vi "Open.vi"   [LabVIEW 2011, in "LMH-Xbox-One-Controller.lvlib"]
uses:
  LMH-Xbox-One-Controller.lvlib
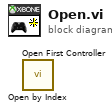
[diagram p0: block diagram]
diagram:
  n1 = call "Open by Index.vi"() -> ()  [unwired: 9 in, 3 out]
  n2 = call "Open First Controller.vi"() -> ()  [unwired: 9 in, 3 out]
